vi "Get_Mode.vi"(6 "error in (no error)":errorcluster, 9 "VISA resource name":refnum<visa-resource-name>="Master_Oscilloscope") -> (0 "error out":errorcluster, 2 "Mode":string[](array[string]), 3 "VISA resource name out":refnum<visa-resource-name>)   [LabVIEW 2020]
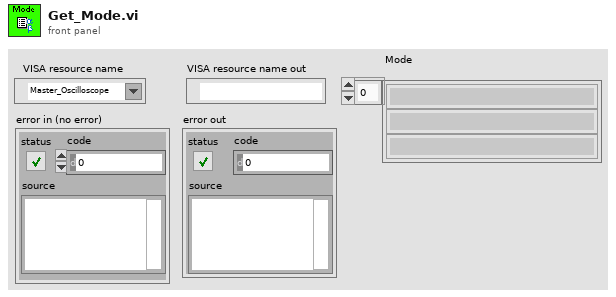
[diagram p1: front panel]
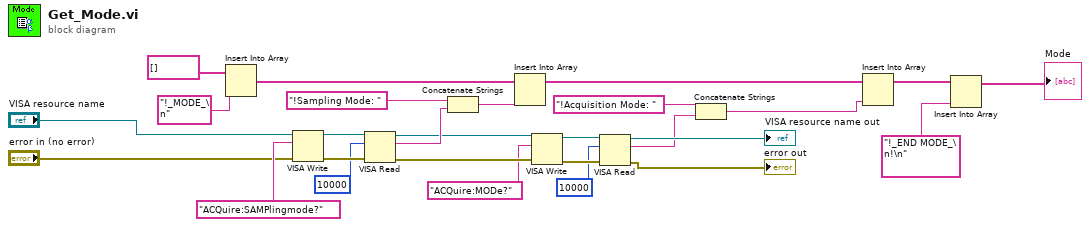
[diagram p0: block diagram]
diagram:
  n1 = Insert Into Array(array=string[] [], new element="!_MODE_\n" ("new element/subarray")) -> (w4:string[])  [unwired: 1 in]
  n2 = VISA Write(VISA resource name="VISA resource name", write buffer="ACQuire:SAMPlingmode?", error in (no error)="error in (no error)") -> (VISA resource name out=w25:refnum<visa-resource-name>, error out=w26:errorcluster)  [unwired: 1 out]
  n3 = VISA Read(VISA resource name=w25, byte count=u32 10000, error in (no error)=w26) -> (VISA resource name out=w17:refnum<visa-resource-name>, read buffer=w20:string, error out=w16:errorcluster)  [unwired: 1 out]
  n4 = Concatenate Strings("!Sampling Mode: ", w20) -> (w19:string)
  n5 = Insert Into Array(array=w4, new element=w19) -> (w18:string[])  [unwired: 1 in]
  n6 = VISA Write(VISA resource name=w17, write buffer="ACQuire:MODe?", error in (no error)=w16) -> (VISA resource name out=w14:refnum<visa-resource-name>, error out=w13:errorcluster)  [unwired: 1 out]
  n7 = VISA Read(VISA resource name=w14, byte count=u32 10000, error in (no error)=w13) -> (VISA resource name out=→"VISA resource name out":refnum<visa-resource-name>, read buffer=w7:string, error out=→"error out":errorcluster)  [unwired: 1 out]
  n8 = Concatenate Strings("!Acquisition Mode: ", w7) -> (w8:string)
  n9 = Insert Into Array(array=w18, new element=w8) -> (w3:string[])  [unwired: 1 in]
  n10 = Insert Into Array(array=w3, new element="!_END MODE_\n!\n" ("new element/subarray")) -> (→"Mode":string[])  [unwired: 1 in]
